vi "CRYCheck Change Before Update.vi"(10 "New Flatten Stimulus Element":string, 11 "Old Flatten Stimulus Element":string) -> (3 "Is Change?":bool)   [LabVIEW 2013]
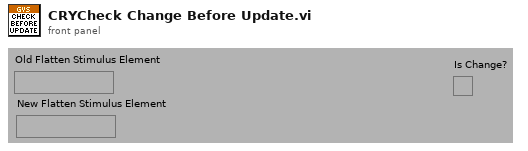
[diagram p1: front panel]
types:
  T1 = typedef "CRYfstepsw.ctl" = cluster{"Level(U)":dbl, "Start Freq(Hz)":dbl, "Stop Freq(Hz)":dbl, "ML val level name":string, "Use ML Val level?":bool, "ML axis":u8, "Steps (#)":i32, "Cycles/step(#)":u32, "Time/step (s)":dbl, "Step Resolution":u16, "unit":u16, "Start Freq Name":string, "Stop Freq Name":string, "Start Freq Axis":u8, "Stop Freq Axis":u8, "Start Freq Flag":string, "Stop Freq Flag":string, "Output Imp":dbl, "Nominal Imp":dbl, "V on DUT":bool}
  T2 = typedef "CRYflogsw.ctl" = cluster{"Level(U)":dbl, "Start Freq(Hz)":dbl, "Stop Freq(Hz)":dbl, "Sweep Rate(s/dec)":dbl, "Use ML Val level?":bool, "ML val level name":string, "ML axis":u8, "TSR params":cluster{"FSamp":dbl, "FStart":dbl, "FStop":dbl, "NOffset":dbl, "MStop":dbl, "MStart":dbl, "NHarm":dbl, "Tsamp":dbl, "Amplit":dbl}, "unit":u16, "Start Freq Name":string, "Stop Freq Name":string, "Start Freq Axis":u8, "Stop Freq Axis":u8, "Start Freq Flag":string, "Stop Freq Flag":string, "Output Imp":dbl, "Nominal Imp":dbl, "V on DUT":bool}
  T3 = typedef "CRYampsw.ctl" = cluster{"Freq(Hz)":dbl, "Steps (#)":i32, "Cycles(#)":u32, "Use ML Val freq?":bool, "ML val freq name":string, "ML axis":u8, "Start Ampl(U)":dbl, "Stop Ampl(U)":dbl, "unit":u16}
  T4 = typedef "CRYwavefile.ctl" = cluster{"Level(U)":dbl, "Wave Path":string, "ML axis":u8, "ML val level name":string, "Use ML Val level?":bool, "wave info":string, "wave time":string, "Peak value4":dbl, "RMS value4":dbl, "wave channel":u16, "unit":u16, "Output Imp":dbl, "Nominal Imp":dbl, "V on DUT":bool}
  T5 = typedef "CRYdcconn.ctl" = cluster{"dc ctrl":u16, "dcmax I":u16, "dc polar":u16, "dc ctrl":u16, "Steps (#)":i32, "Time/step (s)":dbl, "Start Ampl(U)":dbl, "Stop Ampl(U)":dbl, "Level(U)":dbl, "Step Size":dbl}
  T6 = typedef "CRYtwotone.ctl" = cluster{"Steps (#)":i32, "Tone Type":u8, "Freq2(Hz)":dbl, "Time/step (s)":dbl, "Cycles/step (#)":u32, "ML val level name":string, "Use ML Val level?":bool, "Level(U) 2":dbl, "Diff Freq(Hz)":dbl, "ML axis 2":u8, "Diff/Ratio":u8, "Level(U)":dbl, "Stop Freq(Hz)":dbl, "Ratio Val":dbl, "ML val level name 2":string, "Use ML Val level? 2":bool, "ML axis":u8, "Start Freq(Hz)":dbl, "Step Resolution":u16, "Ratio":u16, "TabCtrl6":enum32{"Master Tone", "Slave Tone"}, "unit 1":u16, "unit 2":u16, "Start Freq Name":string, "Stop Freq Name":string, "Start Freq Axis":u8, "Stop Freq Axis":u8, "Start Freq Flag":string, "Stop Freq Flag":string}
  T7 = typedef "CRYmltitone.ctl" = cluster{"Level(U)":dbl, "Min Freq(Hz)":dbl, "Max Freq(Hz)":dbl, "Duration(s)":dbl, "Freq Rounding":bool, "Rounding Val":dbl, "Profile":i32, "ML axis 2":u8, "ML val level name":string, "Use ML Val level?":bool, "ML axis":u8, "Step Resolution":u16, "unit":u16, "Start Freq Name":string, "Stop Freq Name":string, "Start Freq Axis":u8, "Stop Freq Axis":u8, "Start Freq Flag":string, "Stop Freq Flag":string, "Output Imp":dbl, "Nominal Imp":dbl, "V on DUT":bool}
  T8 = typedef "CRYnoise.ctl" = cluster{"Noise Type":u8, "Min Freq(Hz)":dbl, "Max Freq(Hz)":dbl, "Level(U)":dbl, "Duration(s)":dbl, "ML val level name":string, "Use ML Val level?":bool, "ML axis":u8, "unit":u16, "Start Freq Name":string, "Stop Freq Name":string, "Start Freq Axis":u8, "Stop Freq Axis":u8, "Start Freq Flag":string, "Stop Freq Flag":string, "Output Imp":dbl, "Nominal Imp":dbl, "V on DUT":bool}
  T9 = cluster{"fstepsw":T1, "flogsw":T2, "ampsw":T3, "wavefile":T4, "dcconn":T5, "twotone":T6, "mltitone":T7, "noise":T8, "sqwvsw":cluster{"Level(U)":dbl, "Duty Cycle":dbl, "ML val level name":string, "ML axis":u8, "Start Freq(Hz)":u32, "Stop Freq(Hz)":u32, "Use ML Val level?":bool, "Steps (#)":u32, "Cycles/step (#)":u32, "Time/step (s)":dbl, "Step Resolution":u16}, "tnbrst":cluster{"Level(U)":dbl, "ML val level name":string, "ML axis":u8, "Start Freq(Hz)":u32, "Use ML Val level?":bool, "Cycles/step (#)":u32, "Duration(s)":dbl}}
  T10 = cluster{"Data Type":string, "Version":u16, "Dimension":u8}
  T11 = cluster{bool, bool, bool, bool, bool, bool, bool, bool, bool, bool, bool, bool, bool}
  T12 = cluster{bool, bool, bool, bool, bool, bool, bool, bool, bool, bool, bool}
  T13 = cluster{bool, bool, bool, bool, bool, bool, bool, bool}
  T14 = cluster{bool, bool, bool, bool, bool, bool, bool, bool, bool, bool}
  T15 = cluster{bool, bool, bool, bool, bool, bool, bool, bool, bool, bool, bool, bool, bool, bool, bool, bool, bool, bool, bool, bool, bool, bool}
  T16 = cluster{bool, bool, bool, bool, bool, bool, bool, bool, bool, bool, bool, bool}
  T17 = cluster{bool, bool, bool, bool, bool, bool, bool, bool, bool, bool, bool, bool, bool, bool}
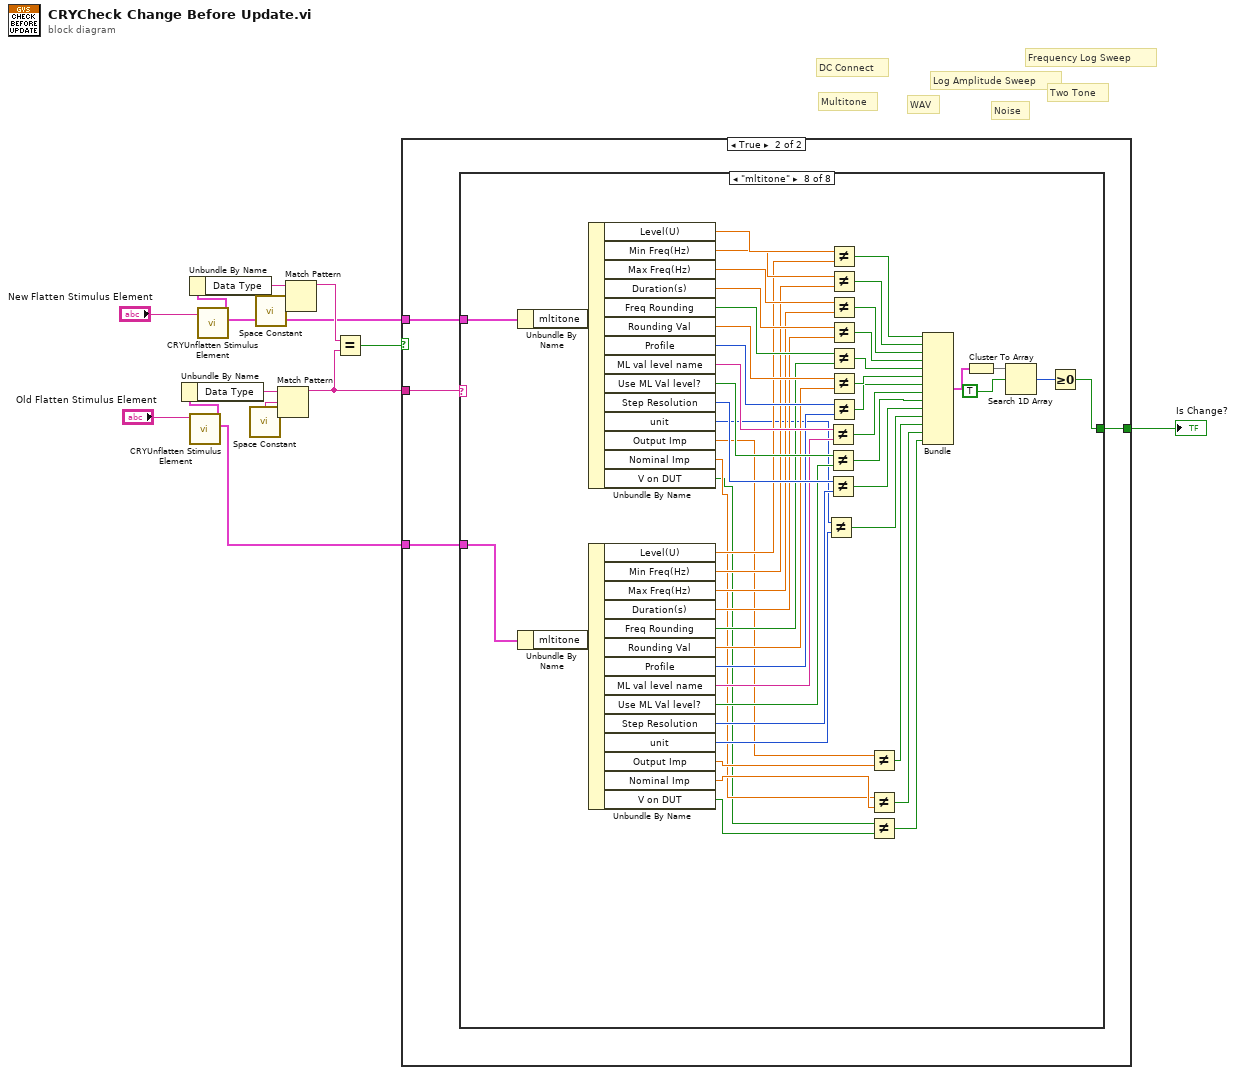
[diagram p0: block diagram]
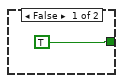
[diagram p2: hidden frame]
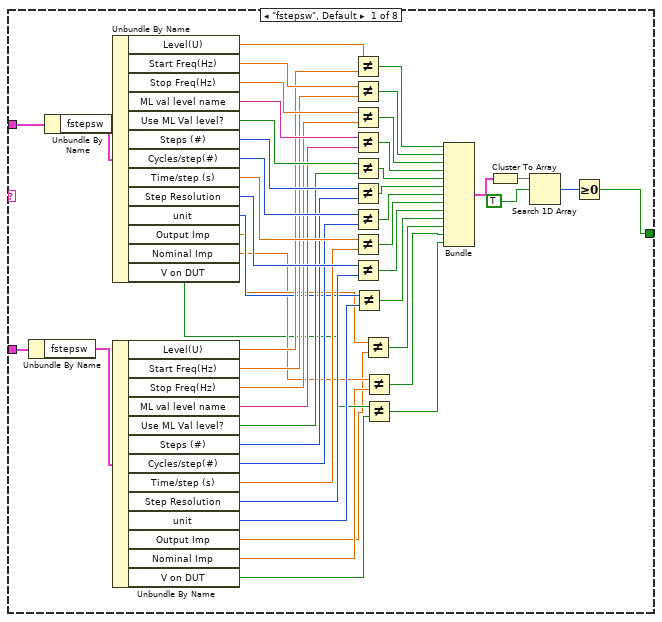
[diagram p3: hidden frame]
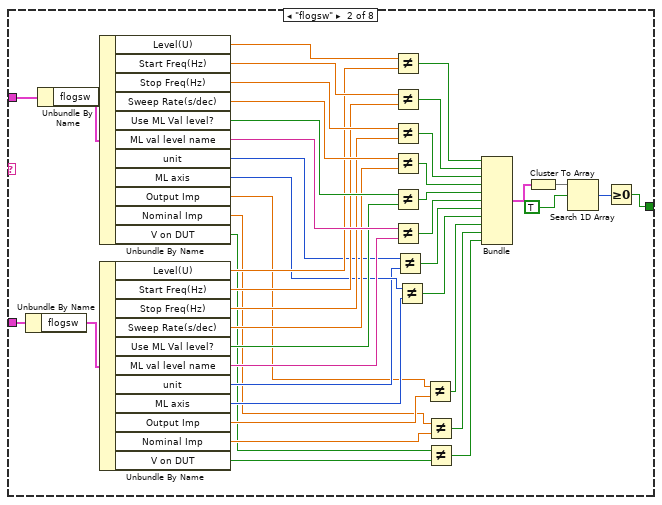
[diagram p4: hidden frame]
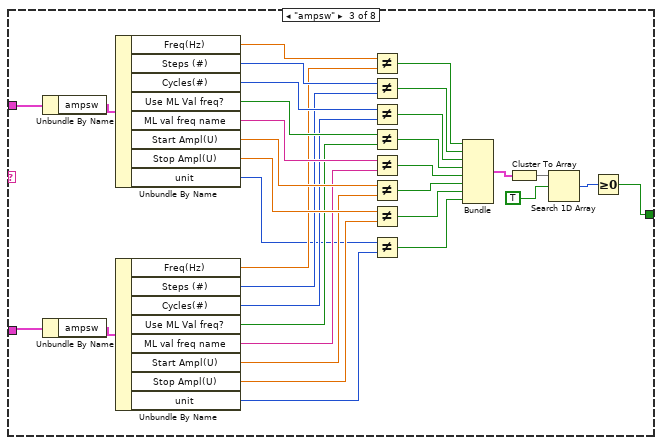
[diagram p5: hidden frame]
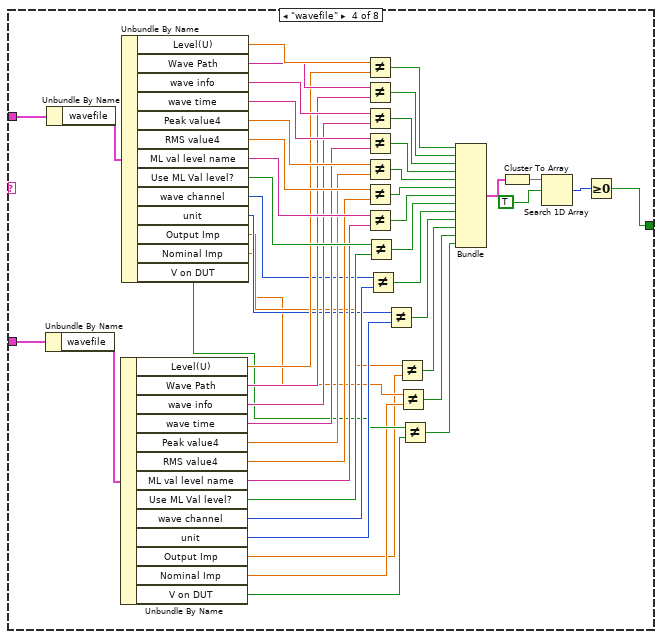
[diagram p6: hidden frame]
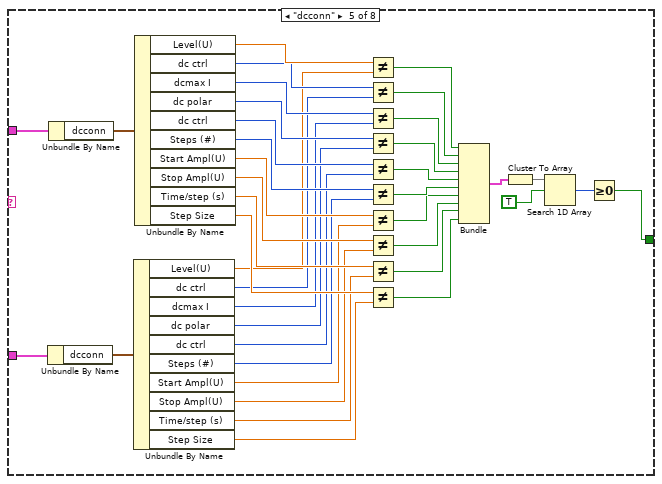
[diagram p7: hidden frame]
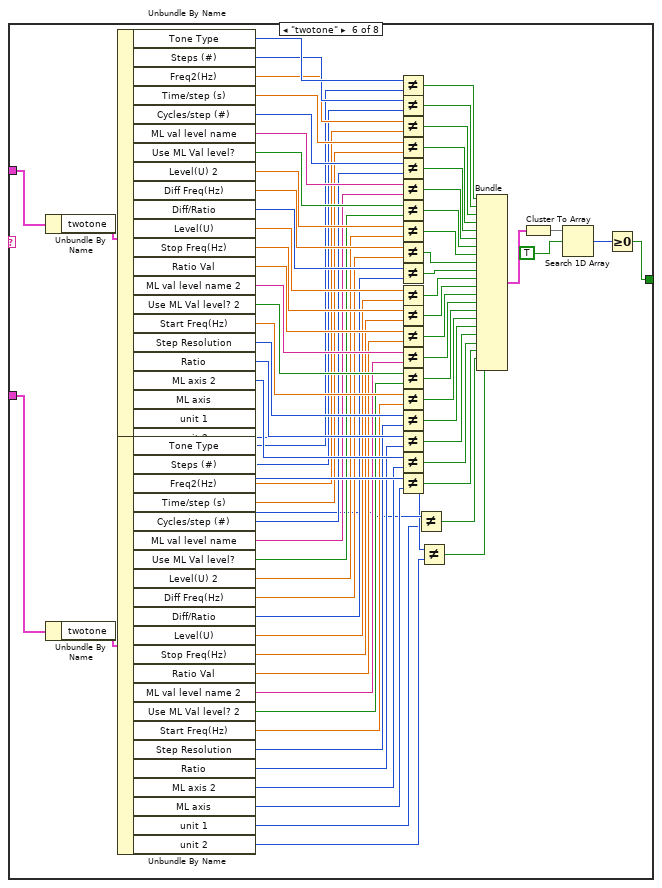
[diagram p8: hidden frame]
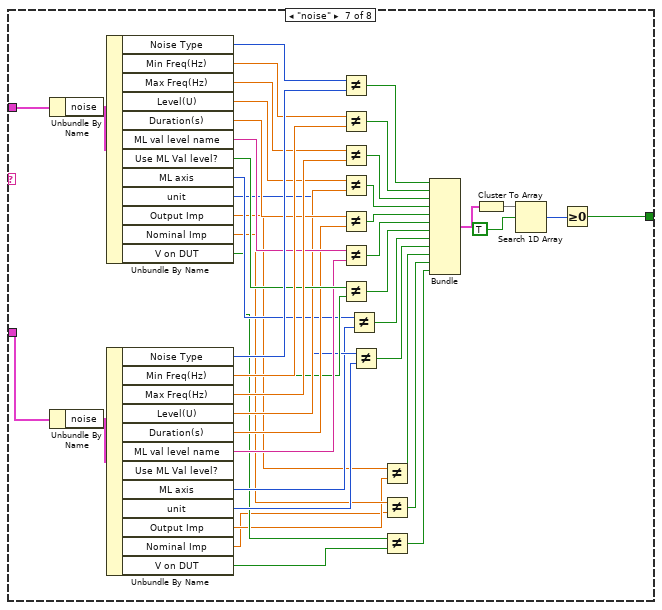
[diagram p9: hidden frame]
diagram:
  # "Multitone"
  # "Noise"
  # "Two Tone"
  # "DC Connect"
  # "WAV"
  # "Log Amplitude Sweep"
  # "Frequency Log Sweep"
  n1 = call "CRYUnflatten Stimulus Element.vi"("Unflatten Stimulus Element setup"="Old Flatten Stimulus Element") -> ("Stimulus Default"=w12:T9, "Header of common"=w13:T10)  [unwired: 1 in, 8 out]
  n2 = Unbundle By Name(w13) -> ("Data Type"=w11:string)
  n3 = call "CRYUnflatten Stimulus Element.vi"("Unflatten Stimulus Element setup"="New Flatten Stimulus Element") -> ("Stimulus Default"=w2:T9, "Header of common"=w7:T10)  [unwired: 1 in, 8 out]
  n4 = Unbundle By Name(w7) -> ("Data Type"=w8:string)
  n5 = call <vilib>:"Space Constant.vi"() -> ("String"=w10:string)
  n6 = call <vilib>:"Space Constant.vi"() -> ("String"=w9:string)
  n7 = Match Pattern(string=w11, regular expression=w10) -> (before substring=w4:string)  [unwired: 4 out]
  n8 = Match Pattern(string=w8, regular expression=w9) -> (before substring=w5:string)  [unwired: 4 out]
  n9 = Equal?(x=w5, y=w4) -> (x = y?=w3:bool)
  n10 = case shown="True" w3 {
    tunnel: w12 -> [_ w19]
    tunnel: w4 -> [_ w18]
    tunnel: w2 -> [_ w17]
    tunnel: [TRUE ("Is Change?") w16] -> w1
    frame False {
    }
    frame True {
      n11 = case shown="\"mltitone\"" w18 {
        tunnel: w19 -> [w67 w109 w141 w189 w228 w303 w348 w399]
        tunnel: w17 -> [w64 w106 w139 w187 w226 w301 w346 w397]
        tunnel: [w32 w83 w113 w158 w191 w236 w320 w362] -> w16
        frame "fstepsw", Default {
          n12 = Unbundle By Name(w67) -> ("fstepsw"=w66:T1)
          n13 = Unbundle By Name(w64) -> ("fstepsw"=w65:T1)
          n14 = Unbundle By Name(w65) -> ("Level(U)"=w50:dbl, "Start Freq(Hz)"=w49:dbl, "Stop Freq(Hz)"=w48:dbl, "ML val level name"=w47:string, "Use ML Val level?"=w46:bool, "Steps (#)"=w45:i32, "Cycles/step(#)"=w44:u32, "Time/step (s)"=w43:dbl, "Step Resolution"=w42:u16, "unit"=w31:u16, "Output Imp"=w25:dbl, "Nominal Imp"=w24:dbl, "V on DUT"=w23:bool)
          n15 = Unbundle By Name(w66) -> ("Level(U)"=w41:dbl, "Start Freq(Hz)"=w40:dbl, "Stop Freq(Hz)"=w39:dbl, "ML val level name"=w38:string, "Use ML Val level?"=w37:bool, "Steps (#)"=w36:i32, "Cycles/step(#)"=w35:u32, "Time/step (s)"=w34:dbl, "Step Resolution"=w33:u16, "unit"=w30:u16, "Output Imp"=w20:dbl, "Nominal Imp"=w21:dbl, "V on DUT"=w22:bool)
          n16 = Not Equal?(x=w50, y=w41) -> (x != y?=w51:bool)
          n17 = Not Equal?(x=w49, y=w40) -> (x != y?=w63:bool)
          n18 = Not Equal?(x=w48, y=w39) -> (x != y?=w62:bool)
          n19 = Not Equal?(x=w47, y=w38) -> (x != y?=w61:bool)
          n20 = Not Equal?(x=w46, y=w37) -> (x != y?=w60:bool)
          n21 = Not Equal?(x=w45, y=w36) -> (x != y?=w59:bool)
          n22 = Not Equal?(x=w44, y=w35) -> (x != y?=w58:bool)
          n23 = Not Equal?(x=w43, y=w34) -> (x != y?=w57:bool)
          n24 = Not Equal?(x=w42, y=w33) -> (x != y?=w52:bool)
          n25 = Not Equal?(x=w31, y=w30) -> (x != y?=w29:bool)
          n26 = Not Equal?(x=w25, y=w20) -> (x != y?=w28:bool)
          n27 = Not Equal?(x=w24, y=w21) -> (x != y?=w27:bool)
          n28 = Not Equal?(x=w23, y=w22) -> (x != y?=w26:bool)
          n29 = Bundle(w51, w63, w62, w61, w60, w59, w58, w57, w52, w29, w28, w27, w26) -> (w56:T11)  [unwired: 1 out]
          n30 = Cluster To Array(cluster=w56) -> (array=w55:bool[])
          n31 = Search 1D Array(1D array=w55, element=TRUE) -> (index of element=w53:i32)  [unwired: 1 out]
          n32 = Greater Or Equal To 0?(x=w53) -> (x >= 0?=w32:bool)
        }
        frame "flogsw" {
          n33 = Unbundle By Name(w109) -> ("flogsw"=w108:T2)
          n34 = Unbundle By Name(w106) -> ("flogsw"=w107:T2)
          n35 = Unbundle By Name(w107) -> ("Level(U)"=w95:dbl, "Start Freq(Hz)"=w94:dbl, "Stop Freq(Hz)"=w93:dbl, "Sweep Rate(s/dec)"=w92:dbl, "Use ML Val level?"=w91:bool, "ML val level name"=w90:string, "unit"=w82:u16, "ML axis"=w81:u8, "Output Imp"=w71:dbl, "Nominal Imp"=w72:dbl, "V on DUT"=w73:bool)
          n36 = Unbundle By Name(w108) -> ("Level(U)"=w89:dbl, "Start Freq(Hz)"=w88:dbl, "Stop Freq(Hz)"=w87:dbl, "Sweep Rate(s/dec)"=w86:dbl, "Use ML Val level?"=w85:bool, "ML val level name"=w84:string, "unit"=w80:u16, "ML axis"=w79:u8, "Output Imp"=w74:dbl, "Nominal Imp"=w75:dbl, "V on DUT"=w76:bool)
          n37 = Not Equal?(x=w95, y=w89) -> (x != y?=w105:bool)
          n38 = Not Equal?(x=w94, y=w88) -> (x != y?=w104:bool)
          n39 = Not Equal?(x=w93, y=w87) -> (x != y?=w103:bool)
          n40 = Not Equal?(x=w92, y=w86) -> (x != y?=w102:bool)
          n41 = Not Equal?(x=w91, y=w85) -> (x != y?=w101:bool)
          n42 = Not Equal?(x=w90, y=w84) -> (x != y?=w100:bool)
          n43 = Not Equal?(x=w82, y=w80) -> (x != y?=w78:bool)
          n44 = Not Equal?(x=w81, y=w79) -> (x != y?=w77:bool)
          n45 = Not Equal?(x=w71, y=w74) -> (x != y?=w70:bool)
          n46 = Not Equal?(x=w72, y=w75) -> (x != y?=w69:bool)
          n47 = Not Equal?(x=w73, y=w76) -> (x != y?=w68:bool)
          n48 = Bundle(w105, w104, w103, w102, w101, w100, w78, w77, w70, w69, w68) -> (w99:T12)  [unwired: 1 out]
          n49 = Cluster To Array(cluster=w99) -> (array=w98:bool[])
          n50 = Search 1D Array(1D array=w98, element=TRUE) -> (index of element=w96:i32)  [unwired: 1 out]
          n51 = Greater Or Equal To 0?(x=w96) -> (x >= 0?=w83:bool)
        }
        frame "ampsw" {
          n52 = Unbundle By Name(w139) -> ("ampsw"=w140:T3)
          n53 = Unbundle By Name(w141) -> ("ampsw"=w142:T3)
          n54 = Unbundle By Name(w140) -> ("Freq(Hz)"=w127:dbl, "Steps (#)"=w126:i32, "Cycles(#)"=w125:u32, "Use ML Val freq?"=w124:bool, "ML val freq name"=w123:string, "Start Ampl(U)"=w122:dbl, "Stop Ampl(U)"=w121:dbl, "unit"=w112:u16)
          n55 = Unbundle By Name(w142) -> ("Freq(Hz)"=w120:dbl, "Steps (#)"=w119:i32, "Cycles(#)"=w118:u32, "Use ML Val freq?"=w117:bool, "ML val freq name"=w116:string, "Start Ampl(U)"=w115:dbl, "Stop Ampl(U)"=w114:dbl, "unit"=w111:u16)
          n56 = Not Equal?(x=w127, y=w120) -> (x != y?=w128:bool)
          n57 = Not Equal?(x=w126, y=w119) -> (x != y?=w138:bool)
          n58 = Not Equal?(x=w125, y=w118) -> (x != y?=w137:bool)
          n59 = Not Equal?(x=w124, y=w117) -> (x != y?=w136:bool)
          n60 = Not Equal?(x=w123, y=w116) -> (x != y?=w135:bool)
          n61 = Not Equal?(x=w122, y=w115) -> (x != y?=w134:bool)
          n62 = Not Equal?(x=w121, y=w114) -> (x != y?=w133:bool)
          n63 = Not Equal?(x=w112, y=w111) -> (x != y?=w110:bool)
          n64 = Bundle(w128, w138, w137, w136, w135, w134, w133, w110) -> (w132:T13)  [unwired: 1 out]
          n65 = Cluster To Array(cluster=w132) -> (array=w131:bool[])
          n66 = Search 1D Array(1D array=w131, element=TRUE) -> (index of element=w129:i32)  [unwired: 1 out]
          n67 = Greater Or Equal To 0?(x=w129) -> (x >= 0?=w113:bool)
        }
        frame "wavefile" {
          n68 = Unbundle By Name(w189) -> ("wavefile"=w190:T4)
          n69 = Unbundle By Name(w187) -> ("wavefile"=w188:T4)
          n70 = Unbundle By Name(w190) -> ("Level(U)"=w166:dbl, "Wave Path"=w165:string, "wave info"=w164:string, "wave time"=w163:string, "Peak value4"=w162:dbl, "RMS value4"=w161:dbl, "ML val level name"=w160:string, "Use ML Val level?"=w159:bool, "wave channel"=w156:u16, "unit"=w153:u16, "Output Imp"=w146:dbl, "Nominal Imp"=w147:dbl, "V on DUT"=w148:bool)
          n71 = Unbundle By Name(w188) -> ("Level(U)"=w175:dbl, "Wave Path"=w173:string, "wave info"=w172:string, "wave time"=w171:string, "Peak value4"=w170:dbl, "RMS value4"=w169:dbl, "ML val level name"=w168:string, "Use ML Val level?"=w167:bool, "wave channel"=w157:u16, "unit"=w154:u16, "Output Imp"=w151:dbl, "Nominal Imp"=w150:dbl, "V on DUT"=w149:bool)
          n72 = Not Equal?(x=w175, y=w166) -> (x != y?=w176:bool)
          n73 = Not Equal?(x=w173, y=w165) -> (x != y?=w186:bool)
          n74 = Not Equal?(x=w172, y=w164) -> (x != y?=w185:bool)
          n75 = Not Equal?(x=w171, y=w163) -> (x != y?=w184:bool)
          n76 = Not Equal?(x=w170, y=w162) -> (x != y?=w183:bool)
          n77 = Not Equal?(x=w169, y=w161) -> (x != y?=w182:bool)
          n78 = Not Equal?(x=w168, y=w160) -> (x != y?=w181:bool)
          n79 = Not Equal?(x=w167, y=w159) -> (x != y?=w174:bool)
          n80 = Not Equal?(x=w157, y=w156) -> (x != y?=w155:bool)
          n81 = Not Equal?(x=w154, y=w153) -> (x != y?=w152:bool)
          n82 = Not Equal?(x=w151, y=w146) -> (x != y?=w145:bool)
          n83 = Not Equal?(x=w150, y=w147) -> (x != y?=w144:bool)
          n84 = Not Equal?(x=w149, y=w148) -> (x != y?=w143:bool)
          n85 = Bundle(w176, w186, w185, w184, w183, w182, w181, w174, w155, w152, w145, w144, w143) -> (w180:T11)  [unwired: 1 out]
          n86 = Cluster To Array(cluster=w180) -> (array=w179:bool[])
          n87 = Search 1D Array(1D array=w179, element=TRUE) -> (index of element=w177:i32)  [unwired: 1 out]
          n88 = Greater Or Equal To 0?(x=w177) -> (x >= 0?=w158:bool)
        }
        frame "dcconn" {
          n89 = Unbundle By Name(w228) -> ("dcconn"=w229:T5)
          n90 = Unbundle By Name(w226) -> ("dcconn"=w227:T5)
          n91 = Unbundle By Name(w229) -> ("Level(U)"=w201:dbl, "dc ctrl"=w200:u16, "dcmax I"=w199:u16, "dc polar"=w198:u16, "dc ctrl"=w197:u16, "Steps (#)"=w196:i32, "Start Ampl(U)"=w195:dbl, "Stop Ampl(U)"=w194:dbl, "Time/step (s)"=w193:dbl, "Step Size"=w192:dbl)
          n92 = Unbundle By Name(w227) -> ("Level(U)"=w211:dbl, "dc ctrl"=w210:u16, "dcmax I"=w209:u16, "dc polar"=w208:u16, "dc ctrl"=w207:u16, "Steps (#)"=w206:i32, "Start Ampl(U)"=w205:dbl, "Stop Ampl(U)"=w204:dbl, "Time/step (s)"=w203:dbl, "Step Size"=w202:dbl)
          n93 = Not Equal?(x=w211, y=w201) -> (x != y?=w212:bool)
          n94 = Not Equal?(x=w210, y=w200) -> (x != y?=w225:bool)
          n95 = Not Equal?(x=w209, y=w199) -> (x != y?=w224:bool)
          n96 = Not Equal?(x=w208, y=w198) -> (x != y?=w223:bool)
          n97 = Not Equal?(x=w207, y=w197) -> (x != y?=w222:bool)
          n98 = Not Equal?(x=w206, y=w196) -> (x != y?=w221:bool)
          n99 = Not Equal?(x=w205, y=w195) -> (x != y?=w220:bool)
          n100 = Not Equal?(x=w204, y=w194) -> (x != y?=w219:bool)
          n101 = Not Equal?(x=w203, y=w193) -> (x != y?=w214:bool)
          n102 = Not Equal?(x=w202, y=w192) -> (x != y?=w213:bool)
          n103 = Bundle(w212, w225, w224, w223, w222, w221, w220, w219, w214, w213) -> (w218:T14)  [unwired: 1 out]
          n104 = Cluster To Array(cluster=w218) -> (array=w217:bool[])
          n105 = Search 1D Array(1D array=w217, element=TRUE) -> (index of element=w215:i32)  [unwired: 1 out]
          n106 = Greater Or Equal To 0?(x=w215) -> (x >= 0?=w191:bool)
        }
        frame "twotone" {
          n107 = Unbundle By Name(w301) -> ("twotone"=w302:T6)
          n108 = Unbundle By Name(w303) -> ("twotone"=w304:T6)
          n109 = Unbundle By Name(w302) -> ("Tone Type"=w286:u8, "Steps (#)"=w275:i32, "Freq2(Hz)"=w274:dbl, "Time/step (s)"=w273:dbl, "Cycles/step (#)"=w272:u32, "ML val level name"=w271:string, "Use ML Val level?"=w270:bool, "Level(U) 2"=w269:dbl, "Diff Freq(Hz)"=w268:dbl, "Diff/Ratio"=w267:u8, "Level(U)"=w266:dbl, "Stop Freq(Hz)"=w265:dbl, "Ratio Val"=w264:dbl, "ML val level name 2"=w263:string, "Use ML Val level? 2"=w262:bool, "Start Freq(Hz)"=w261:dbl, "Step Resolution"=w260:u16, "Ratio"=w259:u16, "ML axis 2"=w258:u8, "ML axis"=w257:u8, "unit 1"=w235:u16, "unit 2"=w234:u16)
          n110 = Unbundle By Name(w304) -> ("Tone Type"=w256:u8, "Steps (#)"=w255:i32, "Freq2(Hz)"=w254:dbl, "Time/step (s)"=w253:dbl, "Cycles/step (#)"=w252:u32, "ML val level name"=w251:string, "Use ML Val level?"=w250:bool, "Level(U) 2"=w249:dbl, "Diff Freq(Hz)"=w248:dbl, "Diff/Ratio"=w247:u8, "Level(U)"=w246:dbl, "Stop Freq(Hz)"=w245:dbl, "Ratio Val"=w244:dbl, "ML val level name 2"=w243:string, "Use ML Val level? 2"=w242:bool, "Start Freq(Hz)"=w241:dbl, "Step Resolution"=w240:u16, "Ratio"=w239:u16, "ML axis 2"=w238:u8, "ML axis"=w237:u8, "unit 1"=w233:u16, "unit 2"=w232:u16)
          n111 = Not Equal?(x=w286, y=w256) -> (x != y?=w287:bool)
          n112 = Not Equal?(x=w275, y=w255) -> (x != y?=w300:bool)
          n113 = Not Equal?(x=w274, y=w254) -> (x != y?=w299:bool)
          n114 = Not Equal?(x=w273, y=w253) -> (x != y?=w298:bool)
          n115 = Not Equal?(x=w272, y=w252) -> (x != y?=w297:bool)
          n116 = Not Equal?(x=w271, y=w251) -> (x != y?=w296:bool)
          n117 = Not Equal?(x=w270, y=w250) -> (x != y?=w295:bool)
          n118 = Not Equal?(x=w269, y=w249) -> (x != y?=w294:bool)
          n119 = Not Equal?(x=w268, y=w248) -> (x != y?=w289:bool)
          n120 = Not Equal?(x=w267, y=w247) -> (x != y?=w288:bool)
          n121 = Not Equal?(x=w266, y=w246) -> (x != y?=w285:bool)
          n122 = Not Equal?(x=w265, y=w245) -> (x != y?=w284:bool)
          n123 = Not Equal?(x=w264, y=w244) -> (x != y?=w283:bool)
          n124 = Not Equal?(x=w263, y=w243) -> (x != y?=w282:bool)
          n125 = Not Equal?(x=w262, y=w242) -> (x != y?=w281:bool)
          n126 = Not Equal?(x=w261, y=w241) -> (x != y?=w280:bool)
          n127 = Not Equal?(x=w260, y=w240) -> (x != y?=w279:bool)
          n128 = Not Equal?(x=w259, y=w239) -> (x != y?=w278:bool)
          n129 = Not Equal?(x=w258, y=w238) -> (x != y?=w277:bool)
          n130 = Not Equal?(x=w257, y=w237) -> (x != y?=w276:bool)
          n131 = Not Equal?(x=w235, y=w233) -> (x != y?=w231:bool)
          n132 = Not Equal?(x=w234, y=w232) -> (x != y?=w230:bool)
          n133 = Bundle(w287, w300, w299, w298, w297, w296, w295, w294, w289, w288, w285, w284, w283, w282, w281, w280, w279, w278, w277, w276, w231, w230) -> (w293:T15)  [unwired: 1 out]
          n134 = Cluster To Array(cluster=w293) -> (array=w292:bool[])
          n135 = Search 1D Array(1D array=w292, element=TRUE) -> (index of element=w290:i32)  [unwired: 1 out]
          n136 = Greater Or Equal To 0?(x=w290) -> (x >= 0?=w236:bool)
        }
        frame "noise" {
          n137 = Unbundle By Name(w346) -> ("noise"=w347:T8)
          n138 = Unbundle By Name(w348) -> ("noise"=w349:T8)
          n139 = Unbundle By Name(w347) -> ("Noise Type"=w345:u8, "Min Freq(Hz)"=w343:dbl, "Max Freq(Hz)"=w341:dbl, "Level(U)"=w339:dbl, "Duration(s)"=w338:dbl, "ML val level name"=w337:string, "Use ML Val level?"=w336:bool, "ML axis"=w319:u8, "unit"=w318:u16, "Output Imp"=w313:dbl, "Nominal Imp"=w312:dbl, "V on DUT"=w311:bool)
          n140 = Unbundle By Name(w349) -> ("Noise Type"=w344:u8, "Min Freq(Hz)"=w342:dbl, "Max Freq(Hz)"=w340:dbl, "Level(U)"=w335:dbl, "Duration(s)"=w334:dbl, "ML val level name"=w333:string, "Use ML Val level?"=w332:bool, "ML axis"=w317:u8, "unit"=w316:u16, "Output Imp"=w310:dbl, "Nominal Imp"=w309:dbl, "V on DUT"=w308:bool)
          n141 = Not Equal?(x=w345, y=w344) -> (x != y?=w331:bool)
          n142 = Not Equal?(x=w343, y=w342) -> (x != y?=w330:bool)
          n143 = Not Equal?(x=w341, y=w340) -> (x != y?=w329:bool)
          n144 = Not Equal?(x=w339, y=w335) -> (x != y?=w328:bool)
          n145 = Not Equal?(x=w338, y=w334) -> (x != y?=w327:bool)
          n146 = Not Equal?(x=w337, y=w333) -> (x != y?=w326:bool)
          n147 = Not Equal?(x=w336, y=w332) -> (x != y?=w325:bool)
          n148 = Not Equal?(x=w319, y=w317) -> (x != y?=w315:bool)
          n149 = Not Equal?(x=w318, y=w316) -> (x != y?=w314:bool)
          n150 = Not Equal?(x=w313, y=w310) -> (x != y?=w307:bool)
          n151 = Not Equal?(x=w312, y=w309) -> (x != y?=w306:bool)
          n152 = Not Equal?(x=w311, y=w308) -> (x != y?=w305:bool)
          n153 = Bundle(w331, w330, w329, w328, w327, w326, w325, w315, w314, w307, w306, w305) -> (w324:T16)  [unwired: 1 out]
          n154 = Cluster To Array(cluster=w324) -> (array=w323:bool[])
          n155 = Search 1D Array(1D array=w323, element=TRUE) -> (index of element=w321:i32)  [unwired: 1 out]
          n156 = Greater Or Equal To 0?(x=w321) -> (x >= 0?=w320:bool)
        }
        frame "mltitone" {
          n157 = Unbundle By Name(w397) -> ("mltitone"=w398:T7)
          n158 = Unbundle By Name(w399) -> ("mltitone"=w400:T7)
          n159 = Unbundle By Name(w398) -> ("Level(U)"=w382:dbl, "Min Freq(Hz)"=w381:dbl, "Max Freq(Hz)"=w380:dbl, "Duration(s)"=w379:dbl, "Freq Rounding"=w378:bool, "Rounding Val"=w377:dbl, "Profile"=w376:i32, "ML val level name"=w375:string, "Use ML Val level?"=w374:bool, "Step Resolution"=w373:u16, "unit"=w361:u16, "Output Imp"=w356:dbl, "Nominal Imp"=w355:dbl, "V on DUT"=w354:bool)
          n160 = Unbundle By Name(w400) -> ("Level(U)"=w372:dbl, "Min Freq(Hz)"=w371:dbl, "Max Freq(Hz)"=w370:dbl, "Duration(s)"=w369:dbl, "Freq Rounding"=w368:bool, "Rounding Val"=w367:dbl, "Profile"=w366:i32, "ML val level name"=w365:string, "Use ML Val level?"=w364:bool, "Step Resolution"=w363:u16, "unit"=w360:u16, "Output Imp"=w358:dbl, "Nominal Imp"=w357:dbl, "V on DUT"=w351:bool)
          n161 = Not Equal?(x=w361, y=w360) -> (x != y?=w359:bool)
          n162 = Not Equal?(x=w375, y=w365) -> (x != y?=w390:bool)
          n163 = Not Equal?(x=w374, y=w364) -> (x != y?=w385:bool)
          n164 = Not Equal?(x=w373, y=w363) -> (x != y?=w384:bool)
          n165 = Not Equal?(x=w382, y=w372) -> (x != y?=w383:bool)
          n166 = Not Equal?(x=w381, y=w371) -> (x != y?=w396:bool)
          n167 = Not Equal?(x=w380, y=w370) -> (x != y?=w395:bool)
          n168 = Not Equal?(x=w379, y=w369) -> (x != y?=w394:bool)
          n169 = Not Equal?(x=w378, y=w368) -> (x != y?=w393:bool)
          n170 = Not Equal?(x=w377, y=w367) -> (x != y?=w392:bool)
          n171 = Not Equal?(x=w376, y=w366) -> (x != y?=w391:bool)
          n172 = Not Equal?(x=w356, y=w358) -> (x != y?=w353:bool)
          n173 = Not Equal?(x=w355, y=w357) -> (x != y?=w352:bool)
          n174 = Not Equal?(x=w354, y=w351) -> (x != y?=w350:bool)
          n175 = Bundle(w383, w396, w395, w394, w393, w392, w391, w390, w385, w384, w359, w353, w352, w350) -> (w389:T17)  [unwired: 1 out]
          n176 = Cluster To Array(cluster=w389) -> (array=w388:bool[])
          n177 = Search 1D Array(1D array=w388, element=TRUE) -> (index of element=w386:i32)  [unwired: 1 out]
          n178 = Greater Or Equal To 0?(x=w386) -> (x >= 0?=w362:bool)
        }
      }
    }
  }
  "Is Change?" <- w1
